vi "Constructor.vi"(8 "ErrorIn":errorcluster, 11 "TAFTraceWindow in":refnum<class "TAFTraceWindow.lvclass">) -> (0 "ErrorOut":errorcluster, 3 "TAFTraceWindow out":refnum<class "TAFTraceWindow.lvclass">)   [LabVIEW 2021]
uses:
  TAFTraceWindow.lvclass
  TAFTraceWindow.lvclass/TAFTraceWindow.ctl
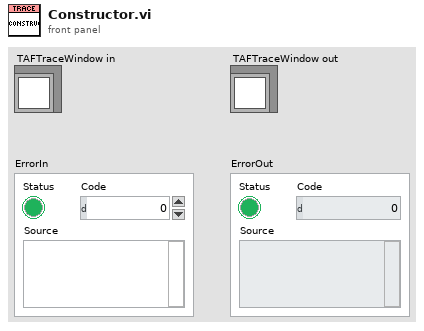
[diagram p1: front panel]
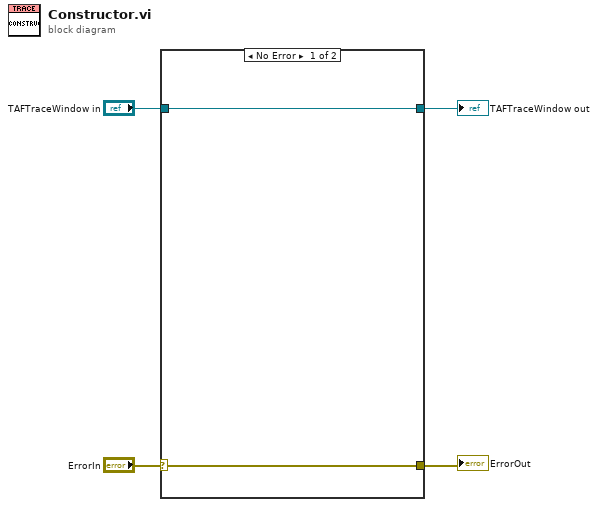
[diagram p0: block diagram]
diagram:
  n1 = case shown="No Error" "ErrorIn" {
    selector: "ErrorIn" -> [w6 w8]
    tunnel: [w6 w8] -> w3
    tunnel: [w5 w7] -> w1
    tunnel: "TAFTraceWindow in" -> [w5 w7]
    frame No Error {
    }
    frame Error {
    }
  }
  "ErrorOut" <- w3
  "TAFTraceWindow out" <- w1
